vi "Read (Waveform)Metodo.vi"(8 "error in (no error)":errorcluster, 9 "Timeout (10000 ms)":u32=10000, 10 "Source (0: Channel 1)":u16(ring) items=["Channel 1", "Channel 2", "Channel 3", "Channel 4", "Math", "Reference A", "Reference B", "Reference C", "Reference D", "FFT"], 11 "Osciloscope in":refnum<class "Osciloscope.lvclass">) -> (0 "error out":errorcluster, 2 "Waveform Data":waveform(dbl)(graph), 3 "Osciloscope out":refnum<class "Osciloscope.lvclass">)   [LabVIEW 2020, in "Osciloscope.lvclass"]
uses:
  Osciloscope.lvclass
  <vilib>/measure/NI_MABase.lvlib
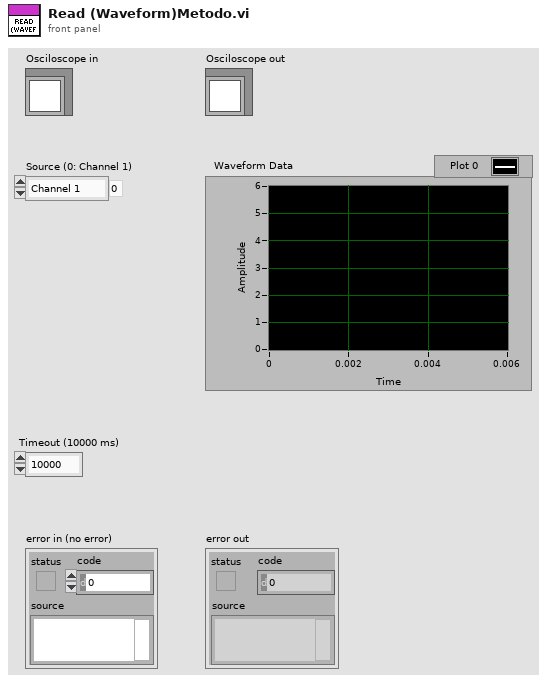
[diagram p1: front panel]
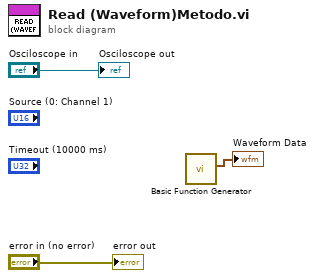
[diagram p0: block diagram]
diagram:
  n1 = call <vilib>:"Basic Function Generator.vi"() -> ("signal out"=→"Waveform Data":waveform(dbl))  [unwired: 9 in, 2 out]
  "Osciloscope out" <- "Osciloscope in"
  "error out" <- "error in (no error)"
